vi "Plot.vi"() -> ()   [LabVIEW 2010]
uses:
  <vilib>/gmath/NI_Gmath.lvlib
panel:
  in  "Plot Legend":i32(listbox)
  in  "AutoScale":bool
  in  "Select All":bool
  out "Waveform Chart":dbl[][](graph)
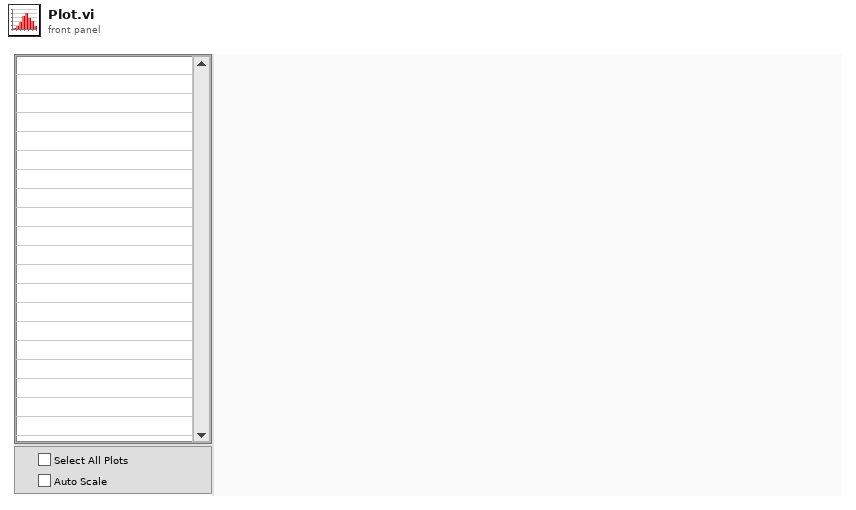
[diagram p1: front panel]
types:
  T1 = cluster{"Error":errorcluster, "PlotNames":string[], "GUIQueue":refnum<queue>, "Telemetry":string, "Format":string, "Equation":string, "IniData":string[][]}
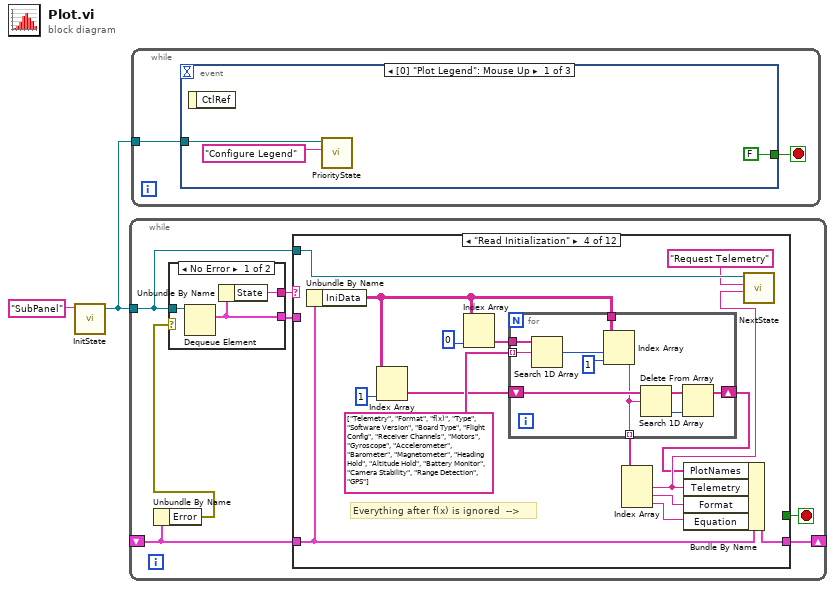
[diagram p0: block diagram]
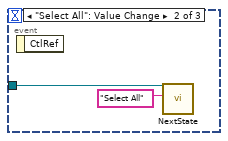
[diagram p2: hidden frame]
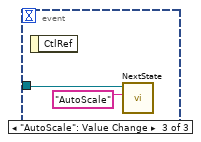
[diagram p3: hidden frame]
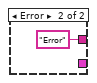
[diagram p4: hidden frame]
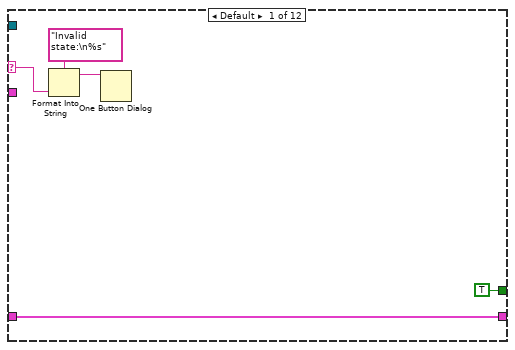
[diagram p5: hidden frame]
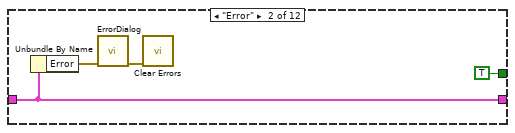
[diagram p6: hidden frame]
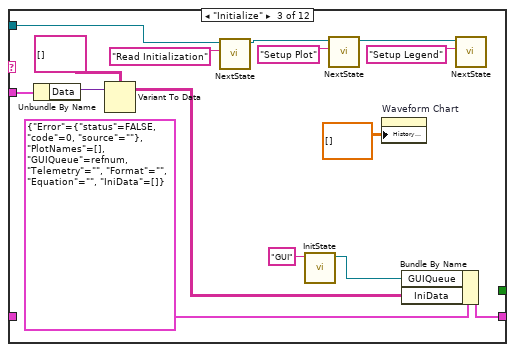
[diagram p7: hidden frame]
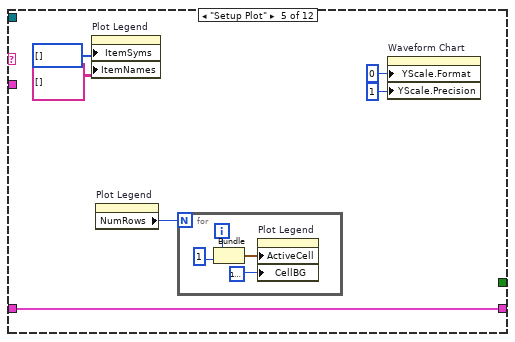
[diagram p8: hidden frame]
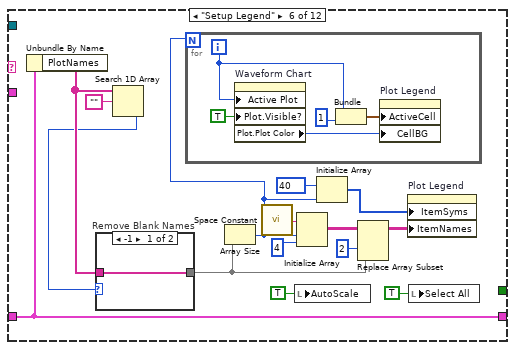
[diagram p9: hidden frame]
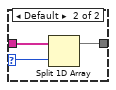
[diagram p10: hidden frame]
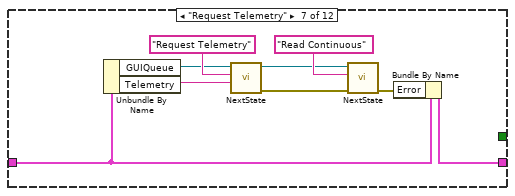
[diagram p11: hidden frame]
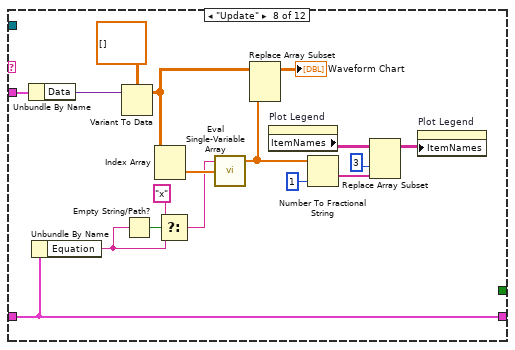
[diagram p12: hidden frame]
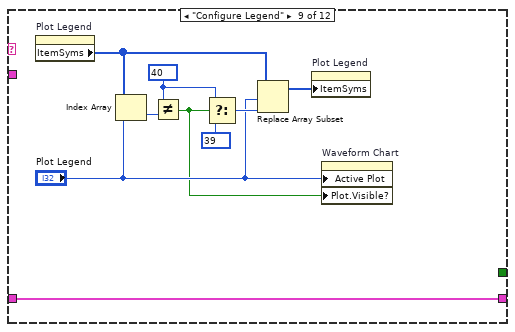
[diagram p13: hidden frame]
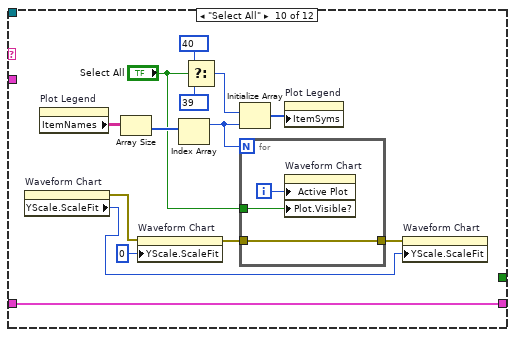
[diagram p14: hidden frame]
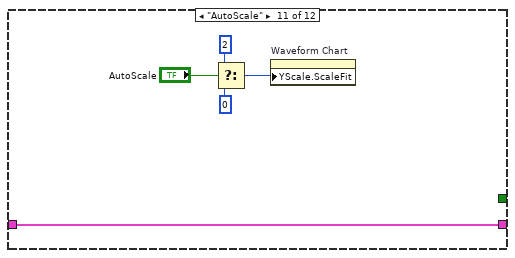
[diagram p15: hidden frame]
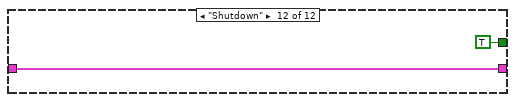
[diagram p16: hidden frame]
diagram:
  n1 = call "InitState.vi"("Name"="SubPanel" ("name (unnamed)")) -> ("Queue Out"=w1:refnum<queue>)  [unwired: 8 in, 1 out]
  n2 = while {
    tunnel: w1 -> [w3]
    shift-right: [w9] -> _
    shift-left: _ -> [w8]
    stop <- w7 stop-if-true
    n3 = Unbundle By Name(w8) -> ("Error"=w6:errorcluster)
    n4 = case shown="No Error" w6 {
      tunnel: [w12 "Error" ("State")] -> w5
      tunnel: [w11 _] -> w4
      tunnel: w3 -> [w10 _]
      frame No Error {
        n5 = Dequeue Element(queue=w10) -> (element=w11:cluster{"State":string, "Data":variant})  [unwired: 2 in, 3 out]
        n6 = Unbundle By Name(w11) -> ("State"=w12:string)
      }
      frame Error {
      }
    }
    n7 = case shown="\"Read Initialization\"" w5 {
      selector: w5 -> [w16 _ _ _ _ _ _ _ _ _ _ _]
      tunnel: w4 -> [_ _ w29 _ _ _ _ w120 _ _ _ _]
      tunnel: w3 -> [_ _ w25 w49 _ _ _ _ _ _ _ _]
      tunnel: [w15 w21 w35 w50 w63 w86 w101 w113 w130 w138 w150 w154] -> w9
      tunnel: w8 -> [w15 w21 _ w51 w63 w86 w103 w113 w130 w138 w150 w154]
      tunnel: [TRUE TRUE _ _ _ _ _ _ _ _ _ TRUE] -> w7
      frame Default {
        n8 = Format Into String(format string="Invalid state:\n%s", w16) -> (resulting string=w17:string)  [unwired: 2 in, 1 out]
        n9 = One Button Dialog(message=w17) -> ()  [unwired: 1 in, 1 out]
      }
      frame "Error" {
        n10 = Unbundle By Name(w21) -> ("Error"=w20:errorcluster)
        n11 = call "ErrorDialog.vi"("error in"=w20) -> ("error out"=w19:errorcluster)  [unwired: 10 in]
        n12 = call <vilib>:"Clear Errors.vi"("error in (no error)"=w19) -> ()  [unwired: 6 in, 1 out]
      }
      frame "Initialize" {
        n13 = Unbundle By Name(w29) -> ("Data"=w28:variant)
        n14 = Variant To Data(Variant=w28, type=string[][] [] ("subarray")) -> (data=w24:string[][])  [unwired: 1 in, 1 out]
        n15 = call "NextState.vi"("State"="Read Initialization", "Queue In"=w25) -> ("Queue Out"=w26:refnum<queue>)  [unwired: 8 in, 1 out]
        n16 = call "InitState.vi"("Name"="GUI") -> ("Queue Out"=w32:refnum<queue>)  [unwired: 8 in, 1 out]
        n17 = call "NextState.vi"("State"="Setup Plot", "Queue In"=w26) -> ("Queue Out"=w31:refnum<queue>)  [unwired: 8 in, 1 out]
        n18 = property on="Waveform Chart" class="WFChart (strict)"("History Data"=dbl[][] []) -> ()  [unwired: 2 in, 2 out]
        n19 = Bundle By Name(cluster=T1 {"Error"={"status"=FALSE, "code"=0, "source"=""}, "PlotNames"=[], "GUIQueue"=refnum, "Telemetry"="", "Format"="", "Equation"="", "IniData"=[]}, "GUIQueue"=w32, "IniData"=w24) -> (w35:T1)
        n20 = call "NextState.vi"("State"="Setup Legend", "Queue In"=w31) -> ()  [unwired: 8 in, 2 out]
      }
      frame "Read Initialization" {
        # "Everything after f(x) is ignored  -->"
        n21 = Unbundle By Name(w51) -> ("IniData"=w44:string[][])
        n22 = Index Array(array=w44, index (col)=1 ("disabled index (col)")) -> (element=w43:string[])  [unwired: 1 in]
        n23 = Index Array(array=w44, index (col)=0 ("index (row)")) -> (element=w46:string[])  [unwired: 1 in]
        n24 = for {
          tunnel: w46 -> [w61]
          tunnel: string[] ["Telemetry", "Format", "f(x)", "Type", "Software Version", "Board Type", "Flight Config", "Receiver Channels", "Motors", "Gyroscope", "Accelerometer", "Barometer", "Magnetometer", "Heading Hold", "Altitude Hold", "Battery Monitor", "Camera Stability", "Range Detection", "GPS"] -> [w56] mode=indexing
          tunnel: w44 -> [w60]
          tunnel: [w53] -> w42 mode=indexing
          shift-right: [w54] -> w38
          shift-left: w43 -> [w57]
          n25 = Search 1D Array(1D array=w61, element=w56) -> (index of element=w58:i32)  [unwired: 1 in]
          n26 = Index Array(array=w60, index (row)=w58, index (col)=1 ("disabled index (col)")) -> (element=w53:string)
          n27 = Search 1D Array(1D array=w57, element=w53) -> (index of element=w55:i32)  [unwired: 1 in]
          n28 = Delete From Array(array=w57, index=w55) -> (array with subset deleted=w54:string[])  [unwired: 1 in, 1 out]
        }
        n29 = Index Array(array=w42) -> (element #1=w39:string, element #2=w41:string, element #3=w40:string)  [unwired: 3 in]
        n30 = Bundle By Name(cluster=w51, "PlotNames"=w38, "Telemetry"=w39, "Format"=w41, "Equation"=w40) -> (w50:T1)
        n31 = call "NextState.vi"("Data"=w39, "State"="Request Telemetry", "Queue In"=w49) -> ()  [unwired: 7 in, 2 out]
      }
      frame "Setup Plot" {
        n32 = property on="Plot Legend" class="MCListbox (strict)"("ItemSyms"=i32[] [] ("Item Symbols"), "ItemNames"=string[][] [] ("Item Names")) -> ()  [unwired: 2 in, 2 out]
        n33 = property on="Plot Legend" class="MCListbox (strict)"() -> ("NumRows"=w62:u32)  [unwired: 2 in, 2 out]
        n34 = for {
          N: w62 -> [_]
          i -> [w69]
          n35 = Bundle(w69, 1) -> (w71:cluster{i32, i32})  [unwired: 1 in]
          n36 = property on="Plot Legend" class="MCListbox (strict)"("ActiveCell"=w71, "CellBG"=u32 16777216) -> ()  [unwired: 2 in, 2 out]
        }
        n37 = property on="Waveform Chart" class="WFChart (strict)"("YScale.Format"=u8 0 ("Y Scale.Display Format:Format"), "YScale.Precision"=u8 1 ("Y Scale.Display Format:Precision")) -> ()  [unwired: 2 in, 2 out]
      }
      frame "Setup Legend" {
        n38 = Unbundle By Name(w86) -> ("PlotNames"=w77:string[])
        n39 = Search 1D Array(1D array=w77, element="") -> (index of element=w74:i32)  [unwired: 1 in]
        n40 = case "Remove Blank Names" shown="-1" w74 {
          selector: w74 -> [_ w88]
          tunnel: w77 -> [w87 w90]
          tunnel: [w87 w89] -> w76
          frame -1 {
          }
          frame Default {
            n41 = Split 1D Array(array=w90, index=w88) -> (first subarray=w89:string[])  [unwired: 1 out]
          }
        }
        n42 = Array Size(array=w76) -> (size(s)=w75:i32)
        n43 = for {
          N: w75 -> [_]
          i -> [w94]
          n44 = property on="Waveform Chart" class="WFChart (strict)"("Active Plot"=w94, "Plot.Visible?"=TRUE ("Plot.Visible")) -> ("Plot.Plot Color"=w92:u32)  [unwired: 2 in, 2 out]
          n45 = Bundle(w94, 1) -> (w93:cluster{i32, i32})  [unwired: 1 in]
          n46 = property on="Plot Legend" class="MCListbox (strict)"("ActiveCell"=w93, "CellBG"=w92) -> ()  [unwired: 2 in, 2 out]
        }
        n47 = call <vilib>:"Space Constant.vi"() -> ("String"=w85:string)
        n48 = local write "AutoScale"(TRUE ("AutoScale")) -> ()
        n49 = Initialize Array(w85, w75, 4 ("dimension size")) -> (w84:string[][])
        n50 = Initialize Array(40, w75) -> (w79:i32[])
        n51 = Replace Array Subset(array=w84, new element=w76, index (col)=2 ("disabled index (col)")) -> (w81:string[][])  [unwired: 1 in]
        n52 = property on="Plot Legend" class="MCListbox (strict)"("ItemSyms"=w79, "ItemNames"=w81) -> ()  [unwired: 2 in, 2 out]
        n53 = local write "Select All"(TRUE ("Select All")) -> ()
      }
      frame "Request Telemetry" {
        n54 = Unbundle By Name(w103) -> ("GUIQueue"=w99:refnum<queue>, "Telemetry"=w98:string)
        n55 = call "NextState.vi"("Data"=w98, "State"="Request Telemetry", "Queue In"=w99) -> ("Error Out"=w96:errorcluster, "Queue Out"=w97:refnum<queue>)  [unwired: 7 in]
        n56 = call "NextState.vi"("Error In"=w96, "State"="Read Continuous", "Queue In"=w97) -> ("Error Out"=w102:errorcluster)  [unwired: 7 in, 1 out]
        n57 = Bundle By Name(cluster=w103, "Error"=w102) -> (w101:T1)
      }
      frame "Update" {
        n58 = Unbundle By Name(w120) -> ("Data"=w119:variant)
        n59 = Unbundle By Name(w113) -> ("Equation"=w111:string)
        n60 = Variant To Data(Variant=w119, type=dbl[][] []) -> (data=w106:dbl[][])  [unwired: 1 in, 1 out]
        n61 = Empty String/Path?(string/path=w111) -> (empty?=w112:bool)
        n62 = Index Array(array=w106) -> (element=w109:dbl[])  [unwired: 2 in]
        n63 = Select(t="x", s=w112, f=w111) -> (s? t:f=w108:string)
        n64 = call <vilib>:"Eval Single-Variable Array.vi"("X Values"=w109, "formula"=w108) -> ("Y Values"=w107:dbl[])  [unwired: 1 in, 1 out]
        n65 = Replace Array Subset(array=w106, new element=w107) -> (→"Waveform Chart":dbl[][])  [unwired: 2 in]
        n66 = property on="Plot Legend" class="MCListbox (strict)"() -> ("ItemNames"=w115:string[][])  [unwired: 2 in, 2 out]
        n67 = Number To Fractional String(number=w107, precision (6)=i16 1) -> (F-format string=w117:string[])  [unwired: 2 in]
        n68 = Replace Array Subset(array=w115, new element=w117, index (col)=3 ("disabled index (col)")) -> (w114:string[][])  [unwired: 1 in]
        n69 = property on="Plot Legend" class="MCListbox (strict)"("ItemNames"=w114) -> ()  [unwired: 2 in, 2 out]
      }
      frame "Configure Legend" {
        w123 = 40
        n70 = property on="Plot Legend" class="MCListbox (strict)"() -> ("ItemSyms"=w128:i32[])  [unwired: 2 in, 2 out]
        n71 = Index Array(array=w128, index="Plot Legend") -> (element=w129:i32)
        n72 = Not Equal?(x=w123, y=w129) -> (x != y?=w122:bool)
        n73 = Select(t=w123, s=w122, f=39) -> (s? t:f=w127:i32)
        n74 = Replace Array Subset(array=w128, new element=w127, index="Plot Legend") -> (w126:i32[])
        n75 = property on="Plot Legend" class="MCListbox (strict)"("ItemSyms"=w126) -> ()  [unwired: 2 in, 2 out]
        n76 = property on="Waveform Chart" class="WFChart (strict)"("Active Plot"="Plot Legend", "Plot.Visible?"=w122) -> ()  [unwired: 2 in, 2 out]
      }
      frame "Select All" {
        n77 = property on="Waveform Chart" class="WFChart (strict)"() -> (error out=w132:errorcluster, "YScale.ScaleFit"=w131:u8)  [unwired: 2 in, 1 out]
        n78 = property on="Plot Legend" class="MCListbox (strict)"() -> ("ItemNames"=w139:string[][])  [unwired: 2 in, 2 out]
        n79 = Array Size(array=w139) -> (size(s)=w144:i32[])
        n80 = property on="Waveform Chart" class="WFChart (strict)"(error in=w132, "YScale.ScaleFit"=u8 0 ("Y Scale.Scale Fit")) -> (error out=w134:errorcluster)  [unwired: 1 in, 1 out]
        n81 = Index Array(array=w144) -> (element=w136:i32)  [unwired: 1 in]
        n82 = Select(t=40, s="Select All", f=39) -> (s? t:f=w141:i32)
        n83 = Initialize Array(w141, w136) -> (w140:i32[])
        n84 = for {
          N: w136 -> [_]
          tunnel: "Select All" -> [w146]
          tunnel: w134 -> [w145]
          tunnel: [w145] -> w133
          i -> [w147]
          n85 = property on="Waveform Chart" class="WFChart (strict)"("Active Plot"=w147, "Plot.Visible?"=w146) -> ()  [unwired: 2 in, 2 out]
        }
        n86 = property on="Plot Legend" class="MCListbox (strict)"("ItemSyms"=w140) -> ()  [unwired: 2 in, 2 out]
        n87 = property on="Waveform Chart" class="WFChart (strict)"(error in=w133, "YScale.ScaleFit"=w131) -> ()  [unwired: 1 in, 2 out]
      }
      frame "AutoScale" {
        n88 = Select(t=u8 2 ("Active Y Scale"), s="AutoScale", f=u8 0 ("Active Y Scale")) -> (s? t:f=w148:u8)
        n89 = property on="Waveform Chart" class="WFChart (strict)"("YScale.ScaleFit"=w148) -> ()  [unwired: 2 in, 2 out]
      }
      frame "Shutdown" {
      }
    }
  }
  n90 = while {
    tunnel: w1 -> [w155]
    stop <- w156 stop-if-true
    n91 = event shown="[0] \"Plot Legend\": Mouse Up" {
      selector: _ -> [_ _ _]
      dyn-events: _ -> [_ _ _]
      timeout: _ -> [_ _ _]
      tunnel: [FALSE _ _] -> w156
      tunnel: w155 -> [w158 w161 w162]
      event "Plot Legend": Mouse Up {
        n92 = event-data() -> ()  [unwired: 1 in, 1 out]
        n93 = call "PriorityState.vi"("State"="Configure Legend", "Queue In"=w158) -> ()  [unwired: 8 in, 2 out]
      }
      event "Select All": Value Change {
        n94 = event-data() -> ()  [unwired: 1 in, 1 out]
        n95 = call "NextState.vi"("State"="Select All", "Queue In"=w161) -> ()  [unwired: 8 in, 2 out]
      }
      event "AutoScale": Value Change {
        n96 = event-data() -> ()  [unwired: 1 in, 1 out]
        n97 = call "NextState.vi"("State"="AutoScale", "Queue In"=w162) -> ()  [unwired: 8 in, 2 out]
      }
    }
  }
